vi "acquireORCAImageHDRwRaw.vi"(3 "Average":i32=1, 4 "Exposure Array":dbl[](array[numeric])) -> (0 "imgHDRRaw":dbl[][](array[numeric]), 2 "imgHDR":dbl[][](array[numeric]))   [LabVIEW 2016]
uses:
  <vilib>/Utility/error.llb/DialogType.ctl
  IVCCM Software V2/LabView Library/GlobalVariables.vi
panel:
  in  "milliseconds to wait":u32=100
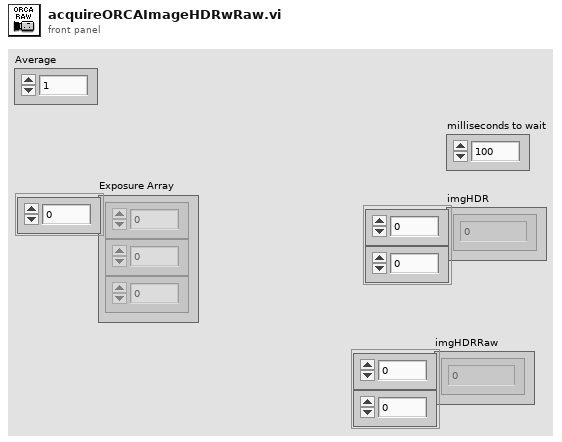
[diagram p1: front panel]
types:
  T1 = cluster{"height":u32, "width":u32, "datatype":u32}
  T2 = typedef "DialogType.ctl" = u16
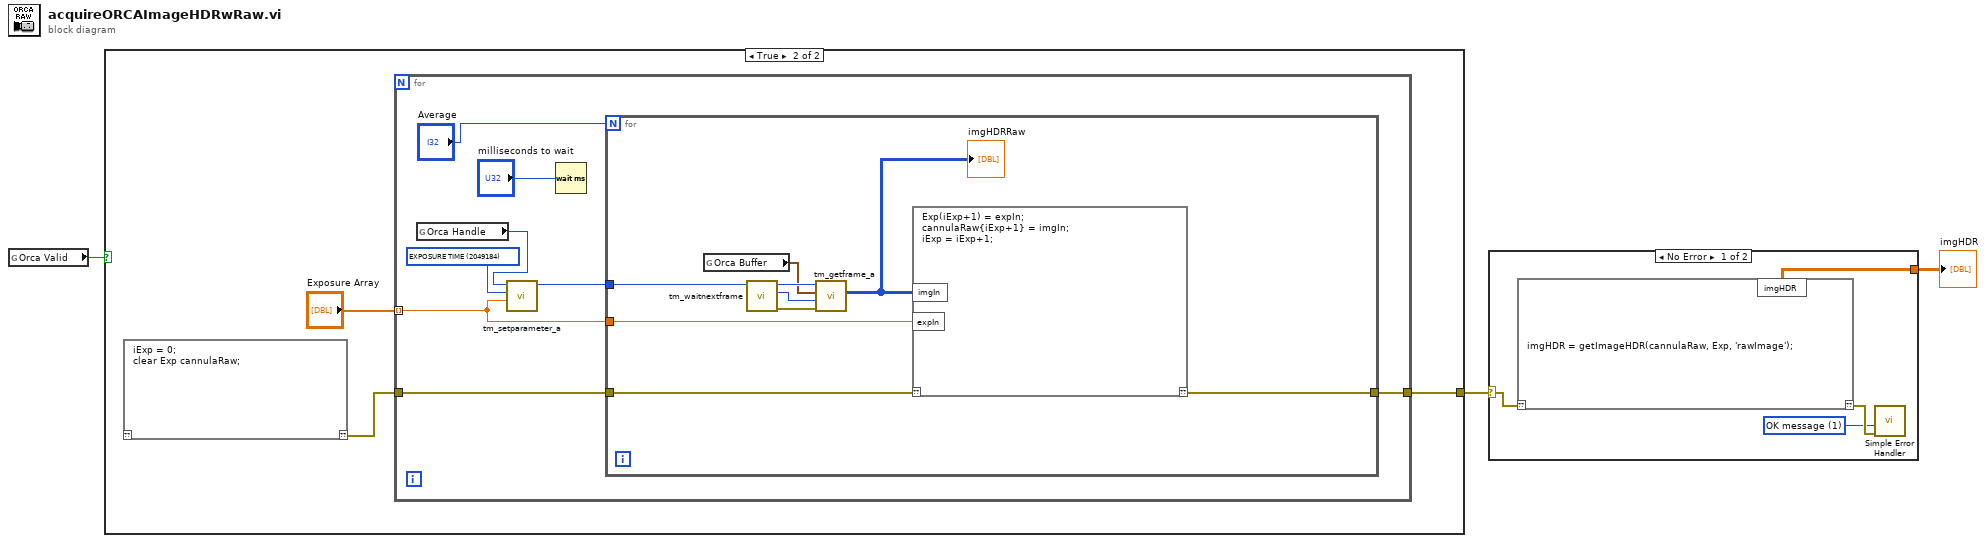
[diagram p0: block diagram]
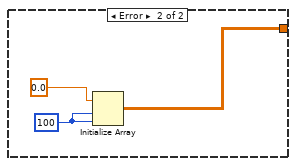
[diagram p2: hidden frame]
diagram:
  n1 = global read "GlobalVariables.vi" "Orca Valid"() -> (w1:bool)
  n2 = case shown="True" w1 {
    tunnel: [_ w4] -> w2
    frame False {
    }
    frame True {
      n3 = script code="iExp = 0;\nclear Exp cannulaRaw;"() -> ("??"=w5:errorcluster)  [unwired: 1 in]
      n4 = for {
        tunnel: "Exposure Array" -> [w13] mode=indexing
        tunnel: w5 -> [w10]
        tunnel: [w9] -> w4
        w11 = u32 2049184 items=["SENSOR MODE"=4212128, "CCD MODE"=4212384, "READOUT MODE"=4211872, "ACTIVE VIEW INDEX"=4343136, "BITS PER CHANNEL"=4342976, "IMAGE PIXEL TYPE"=4343296, "BINNING"=4215968, "EXPOSURE TIME"=2049184, "CONTRAST GAIN"=3163312, "CONTRAST OFFSET"=3163328, "LIGHT MODE"=2114720, "SENSITIVITY"=2114992, "PHOTON IMAGING MODE"=2115200, "HIGH DYNAMIC RANGE MODE"=3163360, "WHITE BALANCE"=3163568, "TEMPERATURE"=2115232, "TEMPERATURE TARGET"=2115264, "SENSOR COOLER FAN"=2115296, "LINEBUNDLE HEIGHT"=4212192, "MECHANICAL SHUTTER"=2115488, "BACK FOCUS POSITION"=8422304, "TRIGGER CONNECTOR"=1066432, "TRIGGER SOURCE"=1066144, "OUTPUT TRIGGER SOURCE"=1852576, "TRIGGER GLOBAL EXPOSURE"=2049680, "FIRST TRIGGER BEHAVIOR"=2049696, "CHANNEL SYNC"=1852352, "READOUT DIRECTION"=4211904, "PRE HSYNC COUNT"=1852704, "INTERNAL LINE SPEED"=4226000, "INTERNAL LINE INTERVAL"=4226016] ("Parameter")
        n5 = global read "GlobalVariables.vi" "Orca Handle"() -> (w12:u32)
        n6 = call <userlib>:"tm_setparameter_a.vi"("Value in"=w13, "Parameter"=w11, "Handle in"=w12) -> ("Handle out"=w8:u32)  [unwired: 7 in, 1 out]
        n7 = Wait (ms)(milliseconds to wait="milliseconds to wait") -> ()  [unwired: 1 out]
        n8 = for {
          N: "Average" -> [_]
          tunnel: w13 -> [w20]
          tunnel: w8 -> [w19]
          tunnel: w10 -> [w18]
          tunnel: [w17] -> w9
          n9 = global read "GlobalVariables.vi" "Orca Buffer"() -> (w16:T1)
          n10 = call <userlib>:"tm_waitnextframe.vi"("Handle in"=w19) -> ("error out"=w22:errorcluster, "Frame Index"=w21:i32, "Handle out"=w23:u32)  [unwired: 7 in, 1 out]
          n11 = call <userlib>:"tm_getframe_a.vi"("error in (no error)"=w22, "Frame Index"=w21, "Buffer Info"=w16, "Handle in"=w23) -> ("Data 16"=w15:u16[][])  [unwired: 3 in, 4 out]
          "imgHDRRaw" <- w15
          n12 = script code="Exp(iExp+1) = expIn;\ncannulaRaw{iExp+1} = imgIn;\niExp = iExp+1;"("??"=w18, "imgIn"=w15, "expIn"=w20) -> ("??"=w17:errorcluster)
        }
      }
    }
  }
  n13 = case shown="No Error" w2 {
    selector: w2 -> [w24 _]
    tunnel: [w27 w30] -> w3
    frame No Error {
      w25 = T2 1 items=["no dialog", "OK message", "continue or stop message", "OK message + warnings", "continue/stop + warnings"] ("type of dialog (OK msg:1)")
      n14 = script code="imgHDR = getImageHDR(cannulaRaw, Exp, 'rawImage');"("??"=w24) -> ("??"=w26:errorcluster, "imgHDR"=w27:dbl[][])
      n15 = call <vilib>:"Simple Error Handler.vi"("type of dialog (OK msg:1)"=w25, "error in (no error)"=w26) -> ()  [unwired: 3 in, 5 out]
    }
    frame Error {
      w28 = 100 ("dimension size")
      n16 = Initialize Array "Initialize Array"(0.0 ("element"), w28, w28) -> (w30:dbl[][])
    }
  }
  "imgHDR" <- w3
